vi "SerialPort.Config_Port.vi"(8 "error in (no error)":errorcluster, 10 "Com Port":refnum<visa-resource-name>="COM3", 11 "SerialPort in":refnum<class "SerialPort.lvclass">) -> (0 "error out":errorcluster, 3 "SerialPort out":refnum<class "SerialPort.lvclass">)   [LabVIEW 2018, in "SerialPort.lvclass"]
uses:
  SerialPort.lvclass
  SerialPort.lvclass/SerialPort.ctl
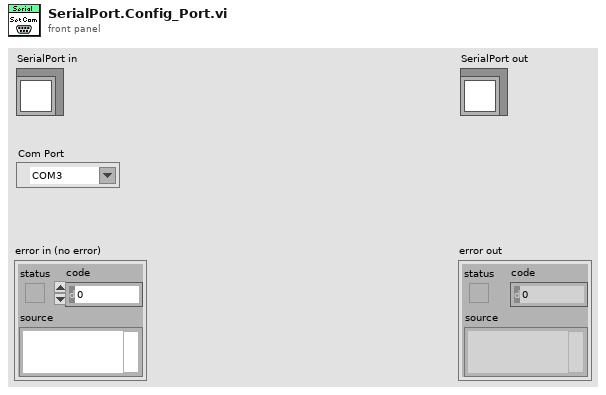
[diagram p1: front panel]
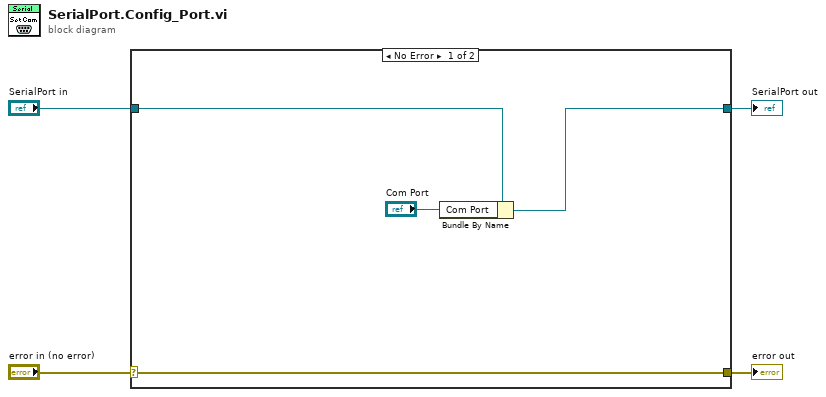
[diagram p0: block diagram]
diagram:
  n1 = case shown="No Error" "error in (no error)" {
    selector: "error in (no error)" -> [w8 w10]
    tunnel: [w8 w10] -> w3
    tunnel: [w6 w9] -> w1
    tunnel: "SerialPort in" -> [w7 w9]
    frame No Error {
      n2 = Bundle By Name(cluster=w7, "Com Port"="Com Port") -> (w6:refnum<class "SerialPort.lvclass">)
    }
    frame Error {
    }
  }
  "error out" <- w3
  "SerialPort out" <- w1
